vi "诊断标定4.vi"(8 "CAN端口":u16(ring), 9 "设备索引号":u16(ring), 10 "CAN卡类型":u32(ring)=4) -> ()   [LabVIEW 2013] (continued)
                                frame True {
                                }
                              }
                              n3940 = local write "正级继电器 8"(w5837) -> ()
                            }
                          }
                        }
                        frame 2 {
                          n3941 = Index Array(array=w5851) -> (element #1=w5850:u8, element #2=w5849:u8, element #3=w5848:u8)  [unwired: 3 in]
                          n3942 = Join Numbers(hi=w5849, lo=w5848) -> ((hi.lo)=w5847:u16)
                          n3943 = case shown="2" w5850 {
                            tunnel: w5851 -> [_ _ _]
                            tunnel: w5847 -> [_ w5855 w5869]
                            tunnel: w5846 -> [_ w5854 _]
                            frame 0, Default {
                              n3944 = local write "继电器超时处理"(FALSE ("继电器超时处理")) -> ()
                            }
                            frame 1 {
                              n3945 = Equal To 0?(x=w5855) -> (x = 0?=w5853:bool)
                              n3946 = case shown="假" w5853 {
                                tunnel: w5855 -> [w5861 _]
                                tunnel: [w5859 "DO控制操作成功!\nDO控制操作成功!\nDO控制操作成功!"] -> _
                                tunnel: w5854 -> [w5858 _]
                                frame False {
                                n3947 = case shown="\"主板\", 默认" w5858 {
                                frame "主板", Default {
                                n3948 = local read "DO1"() -> (w5864:bool)
                                n3949 = Not(x=w5864) -> (.not. x?=w5863:bool)
                                n3950 = local write "DO1"(w5863) -> ()
                                }
                                frame "从板" {
                                n3951 = local read "DO1 2"() -> (w5866:bool)
                                n3952 = Not(x=w5866) -> (.not. x?=w5865:bool)
                                n3953 = local write "DO1 2"(w5865) -> ()
                                }
                                }
                                n3954 = Number To Hexadecimal String(2:w5861) -> (0:w5860:string)  [unwired: 1 out]
                                n3955 = Concatenate Strings("DO控制操作失败,0x" ("消息"), w5860) -> (w5859:string)
                                }
                                frame True {
                                }
                              }
                              n3956 = case shown="\"从板\"" w5854 {
                                tunnel: w5853 -> [w5856 w5857]
                                frame "主板", Default {
                                n3957 = local write "正级继电器 9"(w5856) -> ()
                                }
                                frame "从板" {
                                n3958 = local write "正级继电器 11"(w5857) -> ()
                                }
                              }
                            }
                            frame 2 {
                              n3959 = Equal To 0?(x=w5869) -> (x = 0?=w5868:bool)
                              n3960 = case shown="假" w5868 {
                                tunnel: w5869 -> [w5874 _]
                                tunnel: [w5872 "DO控制操作成功!\nDO控制操作成功!\nDO控制操作成功!"] -> _
                                frame False {
                                n3961 = Number To Hexadecimal String(2:w5874) -> (0:w5873:string)  [unwired: 1 out]
                                n3962 = local read "DO2"() -> (w5871:bool)
                                n3963 = Not(x=w5871) -> (.not. x?=w5870:bool)
                                n3964 = Concatenate Strings("DO控制操作失败,0x" ("消息"), w5873) -> (w5872:string)
                                n3965 = local write "DO2"(w5870) -> ()
                                }
                                frame True {
                                }
                              }
                              n3966 = local write "正级继电器 10"(w5868) -> ()
                            }
                          }
                        }
                      }
                      n3967 = local write "消除"(FALSE ("消除")) -> ()
                      n3968 = global write "EV05全局变量1.vi" "流控帧 2"(FALSE ("流控帧 2")) -> ()
                      n3969 = local write "控制1"(FALSE ("控制1")) -> ()
                      "继电器超时处理" <- TRUE ("控制1")
                    }
                  }
                  n3970 = local write "数据读取判定"(FALSE ("数据读取判定")) -> ()
                }
                frame "高压板校正" {
                  n3971 = local read "命令序号"() -> (w5884:u8)
                  n3972 = call "多帧接收机制(EV05).vi"("can卡类型"=w5890, "设备索引号"=w5889, "CAN端口"=w5888, "VCI_Receive"=w5877, "命令"=w5886, "板号"=w5887, "命令序号"=w5884) -> ("错误信号"=w5880:bool, "错误代码"=w5891:i32, "输出数组"=w5885:u8[], "读错误代码"=w5883:u8[], "结束信号"=w5878:bool)  [unwired: 1 in, 7 out]
                  n3973 = local read "控制1"() -> (w5881:bool)
                  n3974 = local write "数据读取判定"(FALSE ("数据读取判定")) -> ()
                  n3975 = And(x=w5881, y=w5878) -> (x .and. y?=w5882:bool)
                  n3976 = case shown="真" w5882 {
                    tunnel: w5892 -> [_ w5896]
                    tunnel: w5891 -> [_ _]
                    tunnel: w5885 -> [_ w5894]
                    tunnel: w5884 -> [_ w5895]
                    tunnel: w5883 -> [_ w5897]
                    tunnel: w5880 -> [_ w5898]
                    frame False {
                    }
                    frame True {
                      n3977 = case shown="假" w5898 {
                        tunnel: w5897 -> [_ w6106]
                        tunnel: w5896 -> [_ _]
                        tunnel: w5895 -> [w5903 _]
                        tunnel: w5894 -> [w5902 _]
                        frame False {
                          n3978 = case shown="1" w5903 {
                            tunnel: w5902 -> [_ w5908 w5941 w5970 w5997 w6024 w6051 w6078]
                            frame 0, Default {
                            }
                            frame 1 {
                              n3979 = for {
                                N: 10 -> [_]
                                tunnel: w5908 -> [w5925]
                                shift-right: [w5912] -> w5906
                                shift-left: string[] [] -> [w5914]
                                i -> [w5911]
                                w5919 = 8 ("索引")
                                w5923 = 2 ("y")
                                n3980 = Multiply(x=w5911, y=w5923) -> (x*y=w5924:i32)
                                n3981 = Array Subset(array=w5925, index=w5924, length=w5923) -> (w5922:u8[])
                                n3982 = Index Array(array=w5922) -> (element #1=w5921:u8, element #2=w5920:u8)  [unwired: 2 in]
                                n3983 = call "二进制解析-8.6.vi"("索引"=w5919, "数值"=w5921) -> ("低位子数组"=w5918:i32[])  [unwired: 1 in, 2 out]
                                n3984 = call "二进制解析-8.6.vi"("索引"=w5919, "数值"=w5920) -> ("低位子数组"=w5917:i32[])  [unwired: 1 in, 2 out]
                                n3985 = Insert Into Array(array=w5918, new element=w5917) -> (w5916:i32[])  [unwired: 1 in]
                                n3986 = case shown="1" w5911 {
                                tunnel: [6 15 7 4 2 0] -> w5910
                                frame 0, Default {
                                }
                                frame 1 {
                                }
                                frame 2 {
                                }
                                frame 3..5 {
                                }
                                frame 7..9 {
                                }
                                frame 6 {
                                }
                                }
                                n3987 = Reverse 1D Array(array=w5916) -> (reversed array=w5915:i32[])
                                n3988 = for {
                                N: w5910 -> [_]
                                tunnel: w5915 -> [w5936] mode=indexing
                                tunnel: [w5932] -> w5913 mode=indexing
                                n3989 = Equal To 0?(x=w5936) -> (x = 0?=w5935:bool)
                                n3990 = Select(t="无", s=w5935, f="故障") -> (s? t:f=w5932:string)
                                }
                                n3991 = Insert Into Array(array=w5914, new element=w5913) -> (w5912:string[])  [unwired: 1 in]
                              }
                              n3992 = call "详细故障分解.vi"("名称"=string[] ["上电自检异常(CellV)", "通讯异常(CellV)", "不更新(CellV)", "未校准(CellV)", "保留", "采样线路断路(CellV)", "18b20上电自检异常(T) ", "18b20通讯异常(T)", "18b20传感器丢失(T)", "18b20传感器无号(T)", "18b20温度异常跳变(T)", "18b20信号线对电源短路(T)", "18b20信号线对地短路(T)", "18b20 CRC校验异常(T)", "NTC上电自检异常(T)", "NTC通讯异常(T)", "NTC传感器丢失(T)", "NTC温度异常跳变(T)", "NTC信号线断路(T)", "NTC信号线对电源短(T)", "NTC信号线对地短路(T)", "上电自检异常(Curr)", "参数异常(Curr)", "不更新(Curr)", "未校准(Curr)", "采样线断开(Curr)", "电流零漂异常(Curr)", "传感器反接(Curr)", "自检异常(iso)", "前端检测电阻损坏(iso)", "不更新(iso)", "未校准(iso)", "上电自检异常(Sumv_in)", "通讯异常(Sumv_in)", "不更新(Sumv_in)", "未校准(Sumv_in)", "上电自检异常(Sumv_out)", "通讯异常(Sumv_out)", "不更新(Sumv_out)", "未校准(Sumv_out)", "系统时钟自检异常(Clock)", "系统时钟未校准(Clock)", "充电均衡模块不能开启", "充电均衡模块不能关闭", "放电均衡模块不能开启", "放电均衡模块不能关闭"], "故障输入口"=w5906) -> ("输出数组"=w5904:string[][])  [unwired: 1 in, 2 out]
                              n3993 = local write "电池故障"(w5904) -> ()
                            }
                            frame 2 {
                              n3994 = for {
                                N: 5 -> [_]
                                tunnel: w5941 -> [w5958]
                                shift-right: [w5945] -> w5939
                                shift-left: string[] [] -> [w5947]
                                i -> [w5943]
                                w5952 = 8 ("索引")
                                w5956 = 2 ("y")
                                n3995 = Multiply(x=w5943, y=w5956) -> (x*y=w5957:i32)
                                n3996 = Array Subset(array=w5958, index=w5957, length=w5956) -> (w5955:u8[])
                                n3997 = Index Array(array=w5955) -> (element #1=w5954:u8, element #2=w5953:u8)  [unwired: 2 in]
                                n3998 = call "二进制解析-8.6.vi"("索引"=w5952, "数值"=w5954) -> ("低位子数组"=w5951:i32[])  [unwired: 1 in, 2 out]
                                n3999 = call "二进制解析-8.6.vi"("索引"=w5952, "数值"=w5953) -> ("低位子数组"=w5950:i32[])  [unwired: 1 in, 2 out]
                                n4000 = Insert Into Array(array=w5951, new element=w5950) -> (w5949:i32[])  [unwired: 1 in]
                                n4001 = case shown="4" w5943 {
                                tunnel: [4 5] -> w5944
                                frame 0, Default {
                                }
                                frame 4 {
                                }
                                }
                                n4002 = Reverse 1D Array(array=w5949) -> (reversed array=w5948:i32[])
                                n4003 = for {
                                N: w5944 -> [_]
                                tunnel: w5948 -> [w5965] mode=indexing
                                tunnel: [w5961] -> w5946 mode=indexing
                                n4004 = Equal To 0?(x=w5965) -> (x = 0?=w5964:bool)
                                n4005 = Select(t="无", s=w5964, f="故障") -> (s? t:f=w5961:string)
                                }
                                n4006 = Insert Into Array(array=w5947, new element=w5946) -> (w5945:string[])  [unwired: 1 in]
                              }
                              n4007 = call "详细故障分解.vi"("名称"=string[] ["自检异常(ee_cpu)", "存储空间满(ee_cpu)", "数据写入失败(ee_cpu)", "数据读取异常(ee_cpu)", "自检异常(ee_ext)", "存储空间满(ee_ext)", "数据写入失败(ee_ext)", "数据读取异常(ee_ext)", "自检异常(flash_ext)", "存储空间满(flash_ext)", "数据写入失败(flash_ext)", "数据读取异常(flash_ext)", "自检异常(flash_cpu)", "存储空间满(flash_cpu)", "数据写入失败(flash_cpu)", "数据读取异常(flash_cpu)", "应用程序异常(cpu)", "应用程序下载异常(cpu)", "AD模块异常(cpu)", "RAM异常(cpu)", "CPU异常下电(cpu)"], "故障输入口"=w5939) -> ("输出数组"=w5937:string[][])  [unwired: 1 in, 2 out]
                              n4008 = local write "电池故障"(w5937) -> ()
                            }
                            frame 3 {
                              n4009 = for {
                                N: 5 -> [_]
                                tunnel: w5970 -> [w5987]
                                shift-right: [w5974] -> w5968
                                shift-left: string[] [] -> [w5976]
                                i -> [w5973]
                                w5981 = 8 ("索引")
                                w5985 = 2 ("y")
                                n4010 = Multiply(x=w5973, y=w5985) -> (x*y=w5986:i32)
                                n4011 = Array Subset(array=w5987, index=w5986, length=w5985) -> (w5984:u8[])
                                n4012 = Index Array(array=w5984) -> (element #1=w5983:u8, element #2=w5982:u8)  [unwired: 2 in]
                                n4013 = call "二进制解析-8.6.vi"("索引"=w5981, "数值"=w5983) -> ("低位子数组"=w5980:i32[])  [unwired: 1 in, 2 out]
                                n4014 = call "二进制解析-8.6.vi"("索引"=w5981, "数值"=w5982) -> ("低位子数组"=w5979:i32[])  [unwired: 1 in, 2 out]
                                n4015 = Insert Into Array(array=w5980, new element=w5979) -> (w5978:i32[])  [unwired: 1 in]
                                n4016 = Reverse 1D Array(array=w5978) -> (reversed array=w5977:i32[])
                                n4017 = for {
                                N: 6 -> [_]
                                tunnel: w5977 -> [w5992] mode=indexing
                                tunnel: [w5988] -> w5975 mode=indexing
                                n4018 = Equal To 0?(x=w5992) -> (x = 0?=w5991:bool)
                                n4019 = Select(t="无", s=w5991, f="故障") -> (s? t:f=w5988:string)
                                }
                                n4020 = Insert Into Array(array=w5976, new element=w5975) -> (w5974:string[])  [unwired: 1 in]
                              }
                              n4021 = call "详细故障分解.vi"("名称"=string[] ["初始化失败(CAN4)", "发送异常(CAN4)", "接收异常(CAN4)", "总线超时(CAN4)", "BUSOFF(CAN4)", "帧格式(CAN4)", "初始化异常(CAN0)", "发送异常(CAN0)", "接收异常(CAN0)", "总线超时(CAN0)", "BUSOFF(CAN0)", "帧格式(CAN0)", "初始化异常(CAN1)", "发送异常(CAN1)", "接收异常(CAN1)", "总线超时(CAN1)", "BUSOFF(CAN1)", "帧格式(CAN1)", "初始化失败(CAN2)", "发送异常(CAN2)", "接收异常(CAN2)", "总线超时(CAN2)", "BUSOFF(CAN2)", "帧格式(CAN2)", "初始化失败(CAN3)", "发送异常(CAN3)", "接收异常(CAN3)", "总线超时(CAN3)", "BUSOFF(CAN3)", "帧格式(CAN3)"], "故障输入口"=w5968) -> ("输出数组"=w5966:string[][])  [unwired: 1 in, 2 out]
                              n4022 = local write "电池故障"(w5966) -> ()
                            }
                            frame 4 {
                              n4023 = for {
                                N: 1 -> [_]
                                tunnel: w5997 -> [w6014]
                                shift-right: [w6001] -> w5995
                                shift-left: string[] [] -> [w6003]
                                i -> [w6000]
                                w6008 = 8 ("索引")
                                w6012 = 2 ("y")
                                n4024 = Multiply(x=w6000, y=w6012) -> (x*y=w6013:i32)
                                n4025 = Array Subset(array=w6014, index=w6013, length=w6012) -> (w6011:u8[])
                                n4026 = Index Array(array=w6011) -> (element #1=w6010:u8, element #2=w6009:u8)  [unwired: 2 in]
                                n4027 = call "二进制解析-8.6.vi"("索引"=w6008, "数值"=w6010) -> ("低位子数组"=w6007:i32[])  [unwired: 1 in, 2 out]
                                n4028 = call "二进制解析-8.6.vi"("索引"=w6008, "数值"=w6009) -> ("低位子数组"=w6006:i32[])  [unwired: 1 in, 2 out]
                                n4029 = Insert Into Array(array=w6007, new element=w6006) -> (w6005:i32[])  [unwired: 1 in]
                                n4030 = Reverse 1D Array(array=w6005) -> (reversed array=w6004:i32[])
                                n4031 = for {
                                N: 4 -> [_]
                                tunnel: w6004 -> [w6019] mode=indexing
                                tunnel: [w6015] -> w6002 mode=indexing
                                n4032 = Equal To 0?(x=w6019) -> (x = 0?=w6018:bool)
                                n4033 = Select(t="无", s=w6018, f="故障") -> (s? t:f=w6015:string)
                                }
                                n4034 = Insert Into Array(array=w6003, new element=w6002) -> (w6001:string[])  [unwired: 1 in]
                              }
                              n4035 = call "详细故障分解.vi"("名称"=string[] ["通讯协议版本不一致(soft)", "系统不同步(soft)", "软件版本不一致(soft)", "同硬件平台不兼容(soft)"], "故障输入口"=w5995) -> ("输出数组"=w5993:string[][])  [unwired: 1 in, 2 out]
                              n4036 = local write "电池故障"(w5993) -> ()
                            }
                            frame 5 {
                              n4037 = for {
                                N: 2 -> [_]
                                tunnel: w6024 -> [w6041]
                                shift-right: [w6028] -> w6022
                                shift-left: string[] [] -> [w6030]
                                i -> [w6027]
                                w6035 = 8 ("索引")
                                w6039 = 2 ("y")
                                n4038 = Multiply(x=w6027, y=w6039) -> (x*y=w6040:i32)
                                n4039 = Array Subset(array=w6041, index=w6040, length=w6039) -> (w6038:u8[])
                                n4040 = Index Array(array=w6038) -> (element #1=w6037:u8, element #2=w6036:u8)  [unwired: 2 in]
                                n4041 = call "二进制解析-8.6.vi"("索引"=w6035, "数值"=w6037) -> ("低位子数组"=w6034:i32[])  [unwired: 1 in, 2 out]
                                n4042 = call "二进制解析-8.6.vi"("索引"=w6035, "数值"=w6036) -> ("低位子数组"=w6033:i32[])  [unwired: 1 in, 2 out]
                                n4043 = Insert Into Array(array=w6034, new element=w6033) -> (w6032:i32[])  [unwired: 1 in]
                                n4044 = Reverse 1D Array(array=w6032) -> (reversed array=w6031:i32[])
                                n4045 = for {
                                N: 4 -> [_]
                                tunnel: w6031 -> [w6046] mode=indexing
                                tunnel: [w6042] -> w6029 mode=indexing
                                n4046 = Equal To 0?(x=w6046) -> (x = 0?=w6045:bool)
                                n4047 = Select(t="无", s=w6045, f="故障") -> (s? t:f=w6042:string)
                                }
                                n4048 = Insert Into Array(array=w6030, new element=w6029) -> (w6028:string[])  [unwired: 1 in]
                              }
                              n4049 = call "详细故障分解.vi"("名称"=string[] ["初始化失败(RS232)", "发送异常(RS232)", "接收异常(RS232)", "总线超时(RS232)", "初始化失败(RS485)", "发送异常(RS485)", "接收异常(RS485)", "总线超时(RS485)"], "故障输入口"=w6022) -> ("输出数组"=w6020:string[][])  [unwired: 1 in, 2 out]
                              n4050 = local write "电池故障"(w6020) -> ()
                            }
                            frame 6 {
                              n4051 = for {
                                N: 2 -> [_]
                                tunnel: w6051 -> [w6068]
                                shift-right: [w6055] -> w6049
                                shift-left: string[] [] -> [w6057]
                                i -> [w6054]
                                w6062 = 8 ("索引")
                                w6066 = 2 ("y")
                                n4052 = Multiply(x=w6054, y=w6066) -> (x*y=w6067:i32)
                                n4053 = Array Subset(array=w6068, index=w6067, length=w6066) -> (w6065:u8[])
                                n4054 = Index Array(array=w6065) -> (element #1=w6064:u8, element #2=w6063:u8)  [unwired: 2 in]
                                n4055 = call "二进制解析-8.6.vi"("索引"=w6062, "数值"=w6064) -> ("低位子数组"=w6061:i32[])  [unwired: 1 in, 2 out]
                                n4056 = call "二进制解析-8.6.vi"("索引"=w6062, "数值"=w6063) -> ("低位子数组"=w6060:i32[])  [unwired: 1 in, 2 out]
                                n4057 = Insert Into Array(array=w6061, new element=w6060) -> (w6059:i32[])  [unwired: 1 in]
                                n4058 = Reverse 1D Array(array=w6059) -> (reversed array=w6058:i32[])
                                n4059 = for {
                                N: 16 -> [_]
                                tunnel: w6058 -> [w6073] mode=indexing
                                tunnel: [w6069] -> w6056 mode=indexing
                                n4060 = Equal To 0?(x=w6073) -> (x = 0?=w6072:bool)
                                n4061 = Select(t="无", s=w6072, f="故障") -> (s? t:f=w6069:string)
                                }
                                n4062 = Insert Into Array(array=w6057, new element=w6056) -> (w6055:string[])  [unwired: 1 in]
                              }
                              n4063 = call "详细故障分解.vi"("名称"=string[] ["DI1对地短", "DI1对电源短", "DI2对地短", "DI2对电源短", "DI3对地短", "DI3对电源短", "DI4对地短", "DI4对电源短", "DI5对地短", "DI5对电源短", "DI6对地短", "DI6对电源短", "DI7对地短", "DI7对电源短", "DI8对地短", "DI8对电源短", "DO1对地短", "DO1对电源短", "DO2对地短", "DO2对电源短", "DO3对地短", "DO3对电源短", "DO4对地短", "DO4对电源短", "DO5对地短", "DO5对电源短", "DO6对地短", "DO6对电源短", "DO7对地短", "DO7对电源短", "DO8对地短", "DO8对电源短"], "故障输入口"=w6049) -> ("输出数组"=w6047:string[][])  [unwired: 1 in, 2 out]
                              n4064 = local write "电池故障"(w6047) -> ()
                            }
                            frame 7 {
                              n4065 = for {
                                N: 2 -> [_]
                                tunnel: w6078 -> [w6095]
                                shift-right: [w6082] -> w6076
                                shift-left: string[] [] -> [w6084]
                                i -> [w6080]
                                w6089 = 8 ("索引")
                                w6093 = 2 ("y")
                                n4066 = Multiply(x=w6080, y=w6093) -> (x*y=w6094:i32)
                                n4067 = Array Subset(array=w6095, index=w6094, length=w6093) -> (w6092:u8[])
                                n4068 = Index Array(array=w6092) -> (element #1=w6091:u8, element #2=w6090:u8)  [unwired: 2 in]
                                n4069 = call "二进制解析-8.6.vi"("索引"=w6089, "数值"=w6091) -> ("低位子数组"=w6088:i32[])  [unwired: 1 in, 2 out]
                                n4070 = call "二进制解析-8.6.vi"("索引"=w6089, "数值"=w6090) -> ("低位子数组"=w6087:i32[])  [unwired: 1 in, 2 out]
                                n4071 = Insert Into Array(array=w6088, new element=w6087) -> (w6086:i32[])  [unwired: 1 in]
                                n4072 = case shown="1" w6080 {
                                tunnel: [4 6] -> w6081
                                frame 0, Default {
                                }
                                frame 1 {
                                }
                                }
                                n4073 = Reverse 1D Array(array=w6086) -> (reversed array=w6085:i32[])
                                n4074 = for {
                                N: w6081 -> [_]
                                tunnel: w6085 -> [w6102] mode=indexing
                                tunnel: [w6098] -> w6083 mode=indexing
                                n4075 = Equal To 0?(x=w6102) -> (x = 0?=w6101:bool)
                                n4076 = Select(t="无", s=w6101, f="故障") -> (s? t:f=w6098:string)
                                }
                                n4077 = Insert Into Array(array=w6084, new element=w6083) -> (w6082:string[])  [unwired: 1 in]
                              }
                              n4078 = call "详细故障分解.vi"("名称"=string[] ["超时(pre-chg)", "后端开路(pre-chg)", "后端短路(pre-chg)", "预充电回路断开(pre-chg)", "正级继电器驱动故障(relay_driver)", "负级继电器驱动故障(relay_driver)", "预充电继电器驱动故障(relay_driver)", "充电继电器驱动故障(relay_driver)", "风机继电器驱动故障(relay_driver)", "加热继电器驱动故障(relay_driver)"], "故障输入口"=w6076) -> ("输出数组"=w6074:string[][])  [unwired: 1 in, 2 out]
                              n4079 = local write "电池故障"(w6074) -> ()
                            }
                          }
                        }
                        frame True {
                          n4080 = Index Array(array=w6106, index #1=0 ("索引"), index #2=1 ("索引")) -> (element #1=w6109:u8, element #2=w6110:u8)
                          n4081 = Join Numbers(hi=w6109, lo=w6110) -> ((hi.lo)=w6108:u16)
                          n4082 = Number To Hexadecimal String(2:w6108) -> (0:w6107:string)  [unwired: 1 out]
                          n4083 = Concatenate Strings("读取错误，代码： " ("字符串"), "0x" ("字符串"), w6107) -> (w6105:string)
                          n4084 = One Button Dialog(message=w6105, button name ("OK")="是" ("按钮名称（“确定”）")) -> ()  [unwired: 1 out]
                        }
                      }
                      n4085 = local write "消除"(FALSE ("消除")) -> ()
                      n4086 = global write "EV05全局变量1.vi" "流控帧 2"(FALSE ("流控帧 2")) -> ()
                      n4087 = local write "控制1"(FALSE ("控制1")) -> ()
                      n4088 = global write "EV05全局变量1.vi" "写入超时"(TRUE ("写入超时")) -> ()
                    }
                  }
                }
              }
            }
          }
        }
      }
    }
  }
  n4089 = while {
    tunnel: w11 -> [w6119]
    tunnel: w10 -> [w6118]
    tunnel: [w6117] -> w7
    tunnel: [w6116] -> w6
    tunnel: w4 -> [_]
    stop <- w6115 stop-if-true
    n4090 = local read "停止"() -> (w6115:bool)
    n4091 = local read "判定3"() -> (w6114:bool)
    n4092 = case shown="真" w6114 {
      tunnel: w6119 -> [w6122 w6126]
      tunnel: w6118 -> [w6121 w6132]
      tunnel: [w6122 w6125] -> w6117
      tunnel: [w6121 w6124] -> w6116
      frame False {
        n4093 = Wait Until Next ms Multiple(millisecond multiple=u32 10 ("毫秒倍数")) -> ()  [unwired: 1 out]
      }
      frame True {
        n4094 = local read "设备索引号"() -> (w6129:u16)
        n4095 = local read "CAN卡类型"() -> (w6130:u32)
        n4096 = local read "CAN端口"() -> (w6128:u16)
        n4097 = call "receiver-8.6.vi"("CAN端口"=w6128, "设备索引号"=w6129, "CAN卡类型"=w6130) -> ("错误输出"=w6131:errorcluster, "输出簇"=w6127:T25, "接收成功"=w6123:bool)  [unwired: 1 in, 3 out]
        n4098 = call <vilib>:"Clear Errors.vi"("error in (no error)"=w6131) -> ()  [unwired: 6 in, 1 out]
        n4099 = case shown="真" w6123 {
          tunnel: w6132 -> [w6133 w6139]
          tunnel: w6127 -> [_ w6138]
          tunnel: w6126 -> [w6134 w6137]
          tunnel: [w6134 w6136] -> w6125
          tunnel: [w6133 w6135] -> w6124
          frame False {
          }
          frame True {
            n4100 = Enqueue Element(queue=w6137, element=w6138, error in (no error)=w6139) -> (queue out=w6136:refnum<queue>, error out=w6135:errorcluster)  [unwired: 2 out]
          }
        }
      }
    }
  }
  n4101 = while {
    tunnel: w11 -> [w6143]
    tunnel: w10 -> [w6141]
    stop <- w6140 stop-if-true
    n4102 = Dequeue Element(queue=w6143, error in (no error)=w6141) -> (element=w6142:T2, error out=w6140:errorcluster)  [unwired: 3 out]
    n4103 = case shown="无错误" w6140 {
      tunnel: w6142 -> [w6146 _]
      frame No Error {
        n4104 = Unbundle(w6146) -> ("return type"=w6145:u32, "pReceive"=w6144:T1)
        n4105 = for {
          N: w6145 -> [_]
          tunnel: w6144 -> [w6148] mode=indexing
          n4106 = Unbundle By Name(w6148) -> ("ID"=w6151:u32, "1"=w6149:u8, "2"=w6147:u8)
          n4107 = call "ID解析.vi"("ID"=w6151) -> ("PDU(1)"=w6150:i32)  [unwired: 10 out]
          n4108 = case shown="18" w6150 {
            tunnel: w6149 -> [_ w6160]
            tunnel: w6148 -> [_ w6157]
            tunnel: w6147 -> [_ w6153]
            frame 0, Default {
            }
            frame 24 {
              n4109 = call "二进制解析-8.6.vi"("索引"=4, "数值"=w6160) -> ("低位子数组"=w6152:i32[], "高位子数组"=w6161:i32[])  [unwired: 2 out]
              n4110 = call "数值二进制转十进制-8.6.vi"("子数组"=w6152) -> ("十进制数值"=w6158:i32)  [unwired: 4 out]
              n4111 = call "数值二进制转十进制-8.6.vi"("子数组"=w6161) -> ("十进制数值"=w6159:i32)  [unwired: 4 out]
              n4112 = case shown="1" w6159 {
                selector: w6159 -> [w6165 w6182 _]
                tunnel: w6158 -> [_ _ w6189]
                tunnel: [w6165 w6182 w6188] -> w6156
                tunnel: w6153 -> [_ w6177 _]
                tunnel: w6152 -> [_ w6176 _]
                frame 0, Default {
                  n4113 = local write "数据读取判定"(TRUE ("数据读取判定")) -> ()
                  n4114 = local write "循环"(1 ("循环")) -> ()
                }
                frame 1 {
                  n4115 = call "二进制解析-8.6.vi"("索引"=8, "数值"=w6177) -> ("低位子数组"=w6179:i32[])  [unwired: 3 out]
                  n4116 = local write "数据读取判定"(TRUE ("数据读取判定")) -> ()
                  n4117 = local write "1"(0 ("1")) -> ()
                  n4118 = Insert Into Array(array=w6176, new element=w6179) -> (w6175:i32[])  [unwired: 1 in]
                  n4119 = call "数值二进制转十进制-8.6.vi"("子数组"=w6175) -> ("十进制数值"=w6174:i32)  [unwired: 4 out]
                  n4120 = Subtract(x=w6174, y=5) -> (x-y=w6172:i32)
                  n4121 = Quotient & Remainder(x=w6172, y=7) -> (x-y*floor(x/y)=w6170:i32, floor(x/y)=w6168:i32)
                  n4122 = Equal To 0?(x=w6170) -> (x = 0?=w6169:bool)
                  n4123 = Increment(x=w6168) -> (x+1=w6167:i32)
                  n4124 = Select(t=w6168, s=w6169, f=w6167) -> (s? t:f=w6166:i32)
                  n4125 = local write "循环"(w6166) -> ()
                }
                frame 2 {
                  w6187 = 16 ("y")
                  n4126 = Increment(x=w6189) -> (x+1=w6186:i32)
                  n4127 = Equal?(x=w6186, y=w6187) -> (x = y?=w6184:bool)
                  n4128 = case shown="真" w6184 {
                    tunnel: "1" -> [_ w6191]
                    frame False {
                    }
                    frame True {
                      n4129 = Increment(x=w6191) -> (x+1=w6190:i32)
                      n4130 = local write "1"(w6190) -> ()
                    }
                  }
                  n4131 = Multiply(x=w6187, y="1") -> (x*y=w6185:i32)
                  n4132 = Add(x=w6186, y=w6185) -> (x+y=w6188:i32)
                }
              }
              n4133 = local read "临时"() -> (w6154:T1)
              n4134 = Replace Array Subset(array=w6154, new element=w6157, index=w6156) -> (→"临时":T1)
            }
          }
        }
      }
      frame Error {
      }
    }
  }
  n4135 = Release Queue(queue=w7, force destroy? (F)=TRUE ("强制销毁？(F)"), error in (no error)=w6) -> (error out=w9:errorcluster)  [unwired: 2 out]
  n4136 = call <vilib>:"Clear Errors.vi"("error in (no error)"=w9) -> ()  [unwired: 7 out]
  n4137 = local write "数据读取判定"(FALSE ("数据读取判定")) -> ()
  n4138 = local write "循环"(1 ("循环")) -> ()
  n4139 = local write "临时"(T1 [{"ID"=0, "TimeStamp"=0, "TimeFlag"=0, "SendType"=0, "RemoteFlag"=0, "ExternFlag"=0, "DataLen"=0, "1"=0, "2"=0, "3"=0, "4"=0, "5"=0, "6"=0, "7"=0, "8"=0, 0, 0, 0}, {"ID"=0, "TimeStamp"=0, "TimeFlag"=0, "SendType"=0, "RemoteFlag"=0, "ExternFlag"=0, "DataLen"=0, "1"=0, "2"=0, "3"=0, "4"=0, "5"=0, "6"=0, "7"=0, "8"=0, 0, 0, 0}, {"ID"=0, "TimeStamp"=0, "TimeFlag"=0, "SendType"=0, "RemoteFlag"=0, "ExternFlag"=0, "DataLen"=0, "1"=0, "2"=0, "3"=0, "4"=0, "5"=0, "6"=0, "7"=0, "8"=0, 0, 0, 0}, {"ID"=0, "TimeStamp"=0, "TimeFlag"=0, "SendType"=0, "RemoteFlag"=0, "ExternFlag"=0, "DataLen"=0, "1"=0, "2"=0, "3"=0, "4"=0, "5"=0, "6"=0, "7"=0, "8"=0, 0, 0, 0}, {"ID"=0, "TimeStamp"=0, "TimeFlag"=0, "SendType"=0, "RemoteFlag"=0, "ExternFlag"=0, "DataLen"=0, "1"=0, "2"=0, "3"=0, "4"=0, "5"=0, "6"=0, "7"=0, "8"=0, 0, 0, 0}, {"ID"=0, "TimeStamp"=0, "TimeFlag"=0, "SendType"=0, "RemoteFlag"=0, "ExternFlag"=0, "DataLen"=0, "1"=0, "2"=0, "3"=0, "4"=0, "5"=0, "6"=0, "7"=0, "8"=0, 0, 0, 0}, {"ID"=0, "TimeStamp"=0, "TimeFlag"=0, "SendType"=0, "RemoteFlag"=0, "ExternFlag"=0, "DataLen"=0, "1"=0, "2"=0, "3"=0, "4"=0, "5"=0, "6"=0, "7"=0, "8"=0, 0, 0, 0}, {"ID"=0, "TimeStamp"=0, "TimeFlag"=0, "SendType"=0, "RemoteFlag"=0, "ExternFlag"=0, "DataLen"=0, "1"=0, "2"=0, "3"=0, "4"=0, "5"=0, "6"=0, "7"=0, "8"=0, 0, 0, 0}, {"ID"=0, "TimeStamp"=0, "TimeFlag"=0, "SendType"=0, "RemoteFlag"=0, "ExternFlag"=0, "DataLen"=0, "1"=0, "2"=0, "3"=0, "4"=0, "5"=0, "6"=0, "7"=0, "8"=0, 0, 0, 0}, {"ID"=0, "TimeStamp"=0, "TimeFlag"=0, "SendType"=0, "RemoteFlag"=0, "ExternFlag"=0, "DataLen"=0, "1"=0, "2"=0, "3"=0, "4"=0, "5"=0, "6"=0, "7"=0, "8"=0, 0, 0, 0}, {"ID"=0, "TimeStamp"=0, "TimeFlag"=0, "SendType"=0, "RemoteFlag"=0, "ExternFlag"=0, "DataLen"=0, "1"=0, "2"=0, "3"=0, "4"=0, "5"=0, "6"=0, "7"=0, "8"=0, 0, 0, 0}, {"ID"=0, "TimeStamp"=0, "TimeFlag"=0, "SendType"=0, "RemoteFlag"=0, "ExternFlag"=0, "DataLen"=0, "1"=0, "2"=0, "3"=0, "4"=0, "5"=0, "6"=0, "7"=0, "8"=0, 0, 0, 0}, {"ID"=0, "TimeStamp"=0, "TimeFlag"=0, "SendType"=0, "RemoteFlag"=0, "ExternFlag"=0, "DataLen"=0, "1"=0, "2"=0, "3"=0, "4"=0, "5"=0, "6"=0, "7"=0, "8"=0, 0, 0, 0}, {"ID"=0, "TimeStamp"=0, "TimeFlag"=0, "SendType"=0, "RemoteFlag"=0, "ExternFlag"=0, "DataLen"=0, "1"=0, "2"=0, "3"=0, "4"=0, "5"=0, "6"=0, "7"=0, "8"=0, 0, 0, 0}, {"ID"=0, "TimeStamp"=0, "TimeFlag"=0, "SendType"=0, "RemoteFlag"=0, "ExternFlag"=0, "DataLen"=0, "1"=0, "2"=0, "3"=0, "4"=0, "5"=0, "6"=0, "7"=0, "8"=0, 0, 0, 0}, {"ID"=0, "TimeStamp"=0, "TimeFlag"=0, "SendType"=0, "RemoteFlag"=0, "ExternFlag"=0, "DataLen"=0, "1"=0, "2"=0, "3"=0, "4"=0, "5"=0, "6"=0, "7"=0, "8"=0, 0, 0, 0}, {"ID"=0, "TimeStamp"=0, "TimeFlag"=0, "SendType"=0, "RemoteFlag"=0, "ExternFlag"=0, "DataLen"=0, "1"=0, "2"=0, "3"=0, "4"=0, "5"=0, "6"=0, "7"=0, "8"=0, 0, 0, 0}, {"ID"=0, "TimeStamp"=0, "TimeFlag"=0, "SendType"=0, "RemoteFlag"=0, "ExternFlag"=0, "DataLen"=0, "1"=0, "2"=0, "3"=0, "4"=0, "5"=0, "6"=0, "7"=0, "8"=0, 0, 0, 0}, {"ID"=0, "TimeStamp"=0, "TimeFlag"=0, "SendType"=0, "RemoteFlag"=0, "ExternFlag"=0, "DataLen"=0, "1"=0, "2"=0, "3"=0, "4"=0, "5"=0, "6"=0, "7"=0, "8"=0, 0, 0, 0}, {"ID"=0, "TimeStamp"=0, "TimeFlag"=0, "SendType"=0, "RemoteFlag"=0, "ExternFlag"=0, "DataLen"=0, "1"=0, "2"=0, "3"=0, "4"=0, "5"=0, "6"=0, "7"=0, "8"=0, 0, 0, 0}, {"ID"=0, "TimeStamp"=0, "TimeFlag"=0, "SendType"=0, "RemoteFlag"=0, "ExternFlag"=0, "DataLen"=0, "1"=0, "2"=0, "3"=0, "4"=0, "5"=0, "6"=0, "7"=0, "8"=0, 0, 0, 0}, {"ID"=0, "TimeStamp"=0, "TimeFlag"=0, "SendType"=0, "RemoteFlag"=0, "ExternFlag"=0, "DataLen"=0, "1"=0, "2"=0, "3"=0, "4"=0, "5"=0, "6"=0, "7"=0, "8"=0, 0, 0, 0}, {"ID"=0, "TimeStamp"=0, "TimeFlag"=0, "SendType"=0, "RemoteFlag"=0, "ExternFlag"=0, "DataLen"=0, "1"=0, "2"=0, "3"=0, "4"=0, "5"=0, "6"=0, "7"=0, "8"=0, 0, 0, 0}, {"ID"=0, "TimeStamp"=0, "TimeFlag"=0, "SendType"=0, "RemoteFlag"=0, "ExternFlag"=0, "DataLen"=0, "1"=0, "2"=0, "3"=0, "4"=0, "5"=0, "6"=0, "7"=0, "8"=0, 0, 0, 0}, {"ID"=0, "TimeStamp"=0, "TimeFlag"=0, "SendType"=0, "RemoteFlag"=0, "ExternFlag"=0, "DataLen"=0, "1"=0, "2"=0, "3"=0, "4"=0, "5"=0, "6"=0, "7"=0, "8"=0, 0, 0, 0}, {"ID"=0, "TimeStamp"=0, "TimeFlag"=0, "SendType"=0, "RemoteFlag"=0, "ExternFlag"=0, "DataLen"=0, "1"=0, "2"=0, "3"=0, "4"=0, "5"=0, "6"=0, "7"=0, "8"=0, 0, 0, 0}, {"ID"=0, "TimeStamp"=0, "TimeFlag"=0, "SendType"=0, "RemoteFlag"=0, "ExternFlag"=0, "DataLen"=0, "1"=0, "2"=0, "3"=0, "4"=0, "5"=0, "6"=0, "7"=0, "8"=0, 0, 0, 0}, {"ID"=0, "TimeStamp"=0, "TimeFlag"=0, "SendType"=0, "RemoteFlag"=0, "ExternFlag"=0, "DataLen"=0, "1"=0, "2"=0, "3"=0, "4"=0, "5"=0, "6"=0, "7"=0, "8"=0, 0, 0, 0}, {"ID"=0, "TimeStamp"=0, "TimeFlag"=0, "SendType"=0, "RemoteFlag"=0, "ExternFlag"=0, "DataLen"=0, "1"=0, "2"=0, "3"=0, "4"=0, "5"=0, "6"=0, "7"=0, "8"=0, 0, 0, 0}, {"ID"=0, "TimeStamp"=0, "TimeFlag"=0, "SendType"=0, "RemoteFlag"=0, "ExternFlag"=0, "DataLen"=0, "1"=0, "2"=0, "3"=0, "4"=0, "5"=0, "6"=0, "7"=0, "8"=0, 0, 0, 0}, {"ID"=0, "TimeStamp"=0, "TimeFlag"=0, "SendType"=0, "RemoteFlag"=0, "ExternFlag"=0, "DataLen"=0, "1"=0, "2"=0, "3"=0, "4"=0, "5"=0, "6"=0, "7"=0, "8"=0, 0, 0, 0}, {"ID"=0, "TimeStamp"=0, "TimeFlag"=0, "SendType"=0, "RemoteFlag"=0, "ExternFlag"=0, "DataLen"=0, "1"=0, "2"=0, "3"=0, "4"=0, "5"=0, "6"=0, "7"=0, "8"=0, 0, 0, 0}, {"ID"=0, "TimeStamp"=0, "TimeFlag"=0, "SendType"=0, "RemoteFlag"=0, "ExternFlag"=0, "DataLen"=0, "1"=0, "2"=0, "3"=0, "4"=0, "5"=0, "6"=0, "7"=0, "8"=0, 0, 0, 0}, {"ID"=0, "TimeStamp"=0, "TimeFlag"=0, "SendType"=0, "RemoteFlag"=0, "ExternFlag"=0, "DataLen"=0, "1"=0, "2"=0, "3"=0, "4"=0, "5"=0, "6"=0, "7"=0, "8"=0, 0, 0, 0}, {"ID"=0, "TimeStamp"=0, "TimeFlag"=0, "SendType"=0, "RemoteFlag"=0, "ExternFlag"=0, "DataLen"=0, "1"=0, "2"=0, "3"=0, "4"=0, "5"=0, "6"=0, "7"=0, "8"=0, 0, 0, 0}, {"ID"=0, "TimeStamp"=0, "TimeFlag"=0, "SendType"=0, "RemoteFlag"=0, "ExternFlag"=0, "DataLen"=0, "1"=0, "2"=0, "3"=0, "4"=0, "5"=0, "6"=0, "7"=0, "8"=0, 0, 0, 0}, {"ID"=0, "TimeStamp"=0, "TimeFlag"=0, "SendType"=0, "RemoteFlag"=0, "ExternFlag"=0, "DataLen"=0, "1"=0, "2"=0, "3"=0, "4"=0, "5"=0, "6"=0, "7"=0, "8"=0, 0, 0, 0}, {"ID"=0, "TimeStamp"=0, "TimeFlag"=0, "SendType"=0, "RemoteFlag"=0, "ExternFlag"=0, "DataLen"=0, "1"=0, "2"=0, "3"=0, "4"=0, "5"=0, "6"=0, "7"=0, "8"=0, 0, 0, 0}, {"ID"=0, "TimeStamp"=0, "TimeFlag"=0, "SendType"=0, "RemoteFlag"=0, "ExternFlag"=0, "DataLen"=0, "1"=0, "2"=0, "3"=0, "4"=0, "5"=0, "6"=0, "7"=0, "8"=0, 0, 0, 0}, {"ID"=0, "TimeStamp"=0, "TimeFlag"=0, "SendType"=0, "RemoteFlag"=0, "ExternFlag"=0, "DataLen"=0, "1"=0, "2"=0, "3"=0, "4"=0, "5"=0, "6"=0, "7"=0, "8"=0, 0, 0, 0}, {"ID"=0, "TimeStamp"=0, "TimeFlag"=0, "SendType"=0, "RemoteFlag"=0, "ExternFlag"=0, "DataLen"=0, "1"=0, "2"=0, "3"=0, "4"=0, "5"=0, "6"=0, "7"=0, "8"=0, 0, 0, 0}, {"ID"=0, "TimeStamp"=0, "TimeFlag"=0, "SendType"=0, "RemoteFlag"=0, "ExternFlag"=0, "DataLen"=0, "1"=0, "2"=0, "3"=0, "4"=0, "5"=0, "6"=0, "7"=0, "8"=0, 0, 0, 0}, {"ID"=0, "TimeStamp"=0, "TimeFlag"=0, "SendType"=0, "RemoteFlag"=0, "ExternFlag"=0, "DataLen"=0, "1"=0, "2"=0, "3"=0, "4"=0, "5"=0, "6"=0, "7"=0, "8"=0, 0, 0, 0}, {"ID"=0, "TimeStamp"=0, "TimeFlag"=0, "SendType"=0, "RemoteFlag"=0, "ExternFlag"=0, "DataLen"=0, "1"=0, "2"=0, "3"=0, "4"=0, "5"=0, "6"=0, "7"=0, "8"=0, 0, 0, 0}, {"ID"=0, "TimeStamp"=0, "TimeFlag"=0, "SendType"=0, "RemoteFlag"=0, "ExternFlag"=0, "DataLen"=0, "1"=0, "2"=0, "3"=0, "4"=0, "5"=0, "6"=0, "7"=0, "8"=0, 0, 0, 0}] ("数组")) -> ()
  n4140 = Release Queue(queue=w15, force destroy? (F)=TRUE ("强制销毁？(F)"), error in (no error)=w14) -> (error out=w12:errorcluster)  [unwired: 2 out]
  n4141 = call <vilib>:"Clear Errors.vi"("error in (no error)"=w12) -> ()  [unwired: 7 out]
